vi "Transfer Files to Target.vi"() -> ()   [LabVIEW 2026]
uses:
  <vilib>/WebDAVClient/Advanced/Put File.vi
  <vilib>/WebDAVClient/NI_WebDAV.lvlib
panel:
  in  "Custom Device Name":string
  in  "Exit":bool
  in  "Transfer":bool
  in  "RT Target Base Folder":string="/c/ni-rt/CustomDeviceTestBench"
  in  "IP Address":string="0.0.0.0"
  in  "Custom Device Test Hooks PPL Path":path
  in  "Custom Device Deployment Hooks PPL Path":path
  in  "Custom Device PPL Path":path
  in  "JSON File Path":path
  # "Host Machine Paths"
  # "Target"
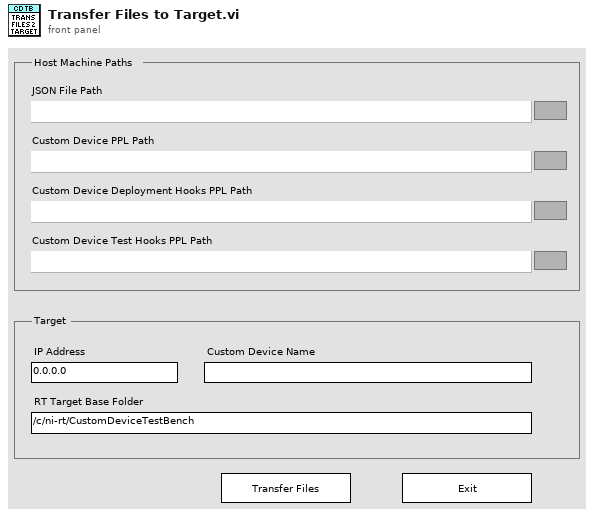
[diagram p1: front panel]
types:
  T1 = typedef "NI_WebDAV.lvlib/SessionHandle.ctl" = refnum<k1>
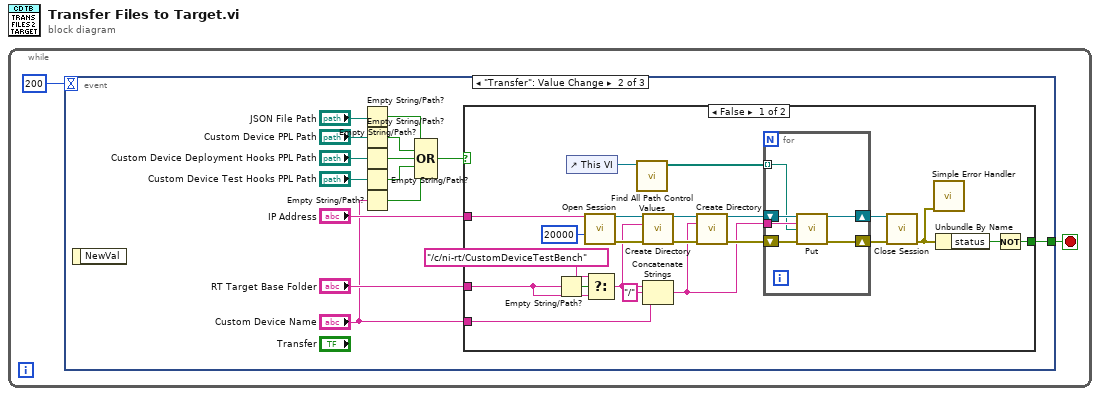
[diagram p0: block diagram]
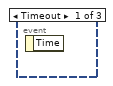
[diagram p2: hidden frame]
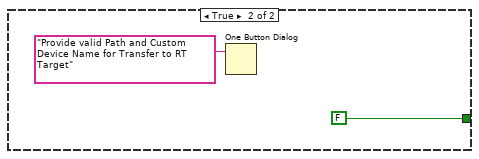
[diagram p3: hidden frame]
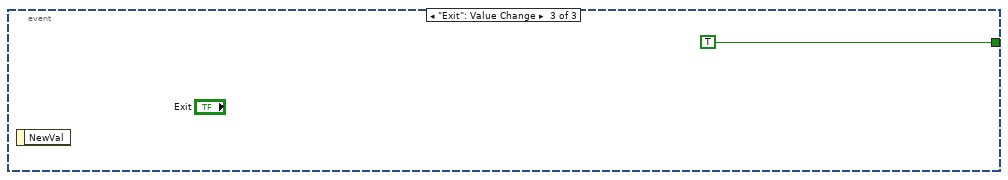
[diagram p4: hidden frame]
diagram:
  n1 = while {
    stop <- w1 stop-if-true
    n2 = event shown="[1] \"Transfer\": Value Change" {
      selector: _ -> [_ _ _]
      dyn-events: _ -> [_ _ _]
      timeout: 200 -> [_ _ _]
      tunnel: [_ w3 TRUE] -> w1
      event Timeout {
        n3 = event-data() -> ()  [unwired: 1 in, 1 out]
      }
      event "Transfer": Value Change {
        n4 = event-data() -> ()  [unwired: 1 in, 1 out]
        n5 = Empty String/Path?(string/path="JSON File Path") -> (empty?=w13:bool)
        n6 = Empty String/Path?(string/path="Custom Device PPL Path") -> (empty?=w12:bool)
        n7 = Empty String/Path?(string/path="Custom Device Deployment Hooks PPL Path") -> (empty?=w9:bool)
        n8 = Empty String/Path?(string/path="Custom Device Test Hooks PPL Path") -> (empty?=w10:bool)
        n9 = Empty String/Path?(string/path="Custom Device Name") -> (empty?=w11:bool)
        n10 = Compound Arithmetic op=OR(w13, w12, w9, w10, w11) -> (w8:bool)
        n11 = case shown="False" w8 {
          tunnel: "IP Address" -> [w35 _]
          tunnel: "RT Target Base Folder" -> [w36 _]
          tunnel: "Custom Device Name" -> [w30 _]
          tunnel: [w18 FALSE] -> w3
          frame False {
            n12 = Empty String/Path?(string/path=w36) -> (empty?=w38:bool)
            n13 = control-ref of="This VI"() -> (w23:refnum<vi>)
            n14 = call <vilib>:"Open Session.vi"("host uri prefix"=w35, "timeout ms"=20000) -> ("session handle out"=w32:T1, "error out"=w33:errorcluster)  [unwired: 12 in]
            n15 = Select(t="/c/ni-rt/CustomDeviceTestBench" ("RT Target Base Folder"), s=w38, f=w36) -> (s? t:f=w29:string)
            n16 = call "Find All Path Control Values.vi"("VI Ref"=w23) -> ("All Paths"=w22:path[])  [unwired: 10 in]
            n17 = call <vilib>:"Create Directory.vi"("session handle"=w32, "relative uri"=w29, "error in (no error)"=w33) -> ("session handle out"=w27:T1, "error out"=w28:errorcluster)  [unwired: 11 in]
            n18 = Concatenate Strings(w29, "/" ("string"), w30) -> (w24:string)
            n19 = call <vilib>:"Create Directory.vi"("session handle"=w27, "relative uri"=w24, "error in (no error)"=w28) -> ("session handle out"=w25:T1, "error out"=w26:errorcluster)  [unwired: 11 in]
            n20 = for {
              tunnel: w24 -> [w42]
              shift-right: [w41] -> w21
              shift-left: w26 -> [w44]
              shift-right: [w40] -> w20
              shift-left: w25 -> [w43]
              tunnel: w22 -> [w39] mode=indexing
              n21 = call-poly <vilib>:"Put.vi"("session handle"=w43, "relative uri"=w42, "local file path"=w39, "error in (no error)"=w44) -> ("session handle out"=w40:T1, "error out"=w41:errorcluster)  [unwired: 9 in, 1 out]
            }
            n22 = call <vilib>:"Close Session.vi"("session handle"=w20, "error in (no error)"=w21) -> ("error out"=w17:errorcluster)  [unwired: 13 in]
            n23 = call <vilib>:"Simple Error Handler.vi"("error in (no error)"=w17) -> ()  [unwired: 4 in, 5 out]
            n24 = Unbundle By Name(w17) -> ("status"=w19:bool)
            n25 = Not(x=w19) -> (.not. x?=w18:bool)
          }
          frame True {
            n26 = One Button Dialog(message="Provide valid Path and Custom Device Name for Transfer to RT Target") -> ()  [unwired: 1 in, 1 out]
          }
        }
      }
      event "Exit": Value Change {
        n27 = event-data() -> ()  [unwired: 1 in, 1 out]
      }
    }
  }
